vi "GetDecorationOwner.vi"(7 "VI Interpreter in":refnum<class "VI Interpreter.lvclass">, 8 "error in":errorcluster, 11 "Decoration in":refnum<class "Decoration.lvclass">) -> (0 "error out":errorcluster, 3 "Decoration out":refnum<class "Decoration.lvclass">, 4 "owner":string, 5 "VI Interpreter out":refnum<class "VI Interpreter.lvclass">)   [LabVIEW 2014, in "PythonConverter_GUI.lvclass"]
uses:
  PythonConverter_GUI.lvclass
  VI Interpreter/Classes/Decoration/Decoration.lvclass
  VI Interpreter/Classes/VI Interpreter/VI Interpreter.lvclass
  VI Interpreter/Classes/Generic/Generic.lvclass/Generic.ctl
  VI Interpreter/Classes/GObject/GObject.lvclass
  VI Interpreter/Classes/Tab/Tab.lvclass
  VI Interpreter/Classes/Generic/Generic.lvclass
  Parsing/Python Functions.lvlib
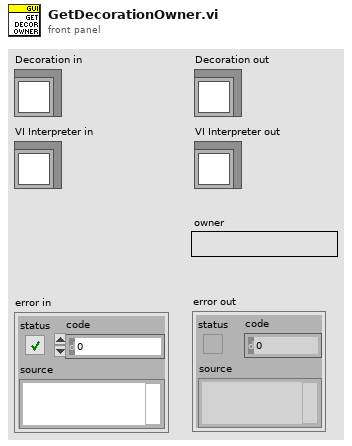
[diagram p1: front panel]
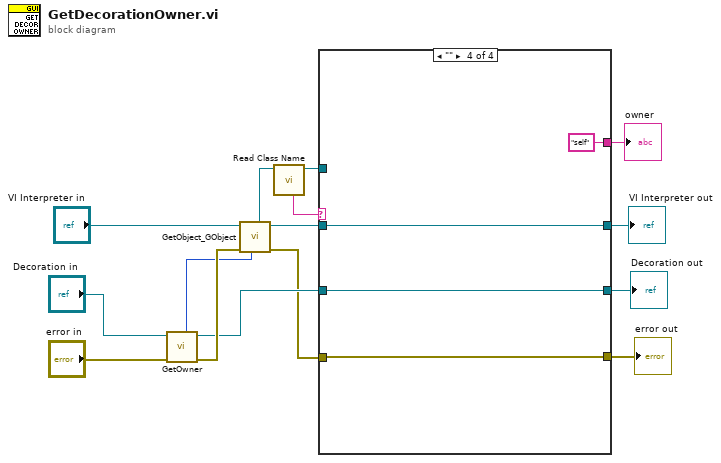
[diagram p0: block diagram]
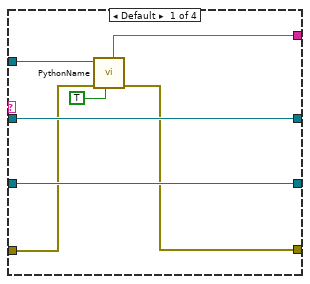
[diagram p2: hidden frame]
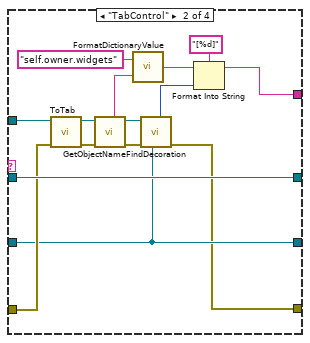
[diagram p3: hidden frame]
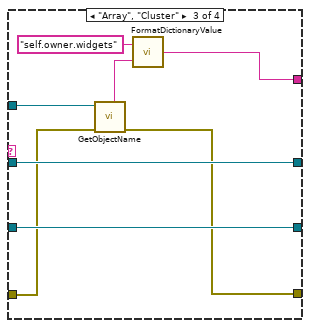
[diagram p4: hidden frame]
diagram:
  n1 = call-dynamic "GetOwner.vi"("error in"="error in", "GObject in"="Decoration in") -> ("error out"=w12:errorcluster, "GObject out"=w4:refnum<class "Decoration.lvclass">, "Owner"=w1:i32)  [unwired: 5 in]
  n2 = call "GetObject_GObject.vi"("UID"=w1, "error in"=w12, "VI Interpreter in"="VI Interpreter in") -> ("error out"=w2:errorcluster, "VI Interpreter out"=w8:refnum<class "VI Interpreter.lvclass">, "GObject"=w11:refnum<class "GObject.lvclass">)  [unwired: 3 in, 1 out]
  n3 = call "Read Class Name.vi"("Generic in"=w11) -> ("Generic out"=w9:refnum<class "GObject.lvclass">, "Class Name"=w10:string)  [unwired: 7 in]
  n4 = case shown="\"\"" w10 {
    tunnel: w9 -> [w22 w36 w40 _]
    tunnel: [w21 w24 w41 "self" ("python object")] -> w7
    tunnel: w8 -> [w19 w37 w45 w48]
    tunnel: [w19 w37 w45 w48] -> w6
    tunnel: [w18 w34 w44 w47] -> w5
    tunnel: w4 -> [w18 w34 w44 w47]
    tunnel: [w17 w23 w38 w46] -> w3
    tunnel: w2 -> [w16 w35 w39 w46]
    frame Default {
      n5 = call-dynamic "PythonName.vi"("add self"=TRUE, "error in"=w16, "GObject in"=w22) -> ("error out"=w17:errorcluster, "name"=w21:string)  [unwired: 5 in, 2 out]
    }
    frame "TabControl" {
      n6 = call "ToTab.vi"("error in"=w35, "Generic in"=w36) -> ("error out"=w32:errorcluster, "Tab out"=w33:refnum<class "Tab.lvclass">)  [unwired: 8 in]
      n7 = call-dynamic "GetObjectName.vi"("error in"=w32, "GObject in"=w33) -> ("error out"=w28:errorcluster, "GObject out"=w29:refnum<class "Tab.lvclass">, "Name"=w31:string)  [unwired: 5 in]
      n8 = call "FormatDictionaryValue.vi"("key"=w31, "dictionary"="self.owner.widgets") -> ("python object"=w26:string)
      n9 = call "FindDecoration.vi"("Decoration in"=w34, "error in"=w28, "Tab in"=w29) -> ("error out"=w23:errorcluster, "Tab index"=w27:i32)  [unwired: 4 in, 1 out]
      n10 = Format Into String(format string="[%d]", initial string=w26, w27) -> (resulting string=w24:string)  [unwired: 1 in, 1 out]
    }
    frame "Array", "Cluster" {
      n11 = call-dynamic "GetObjectName.vi"("error in"=w39, "GObject in"=w40) -> ("error out"=w38:errorcluster, "Name"=w43:string)  [unwired: 5 in, 1 out]
      n12 = call "FormatDictionaryValue.vi"("key"=w43, "dictionary"="self.owner.widgets") -> ("python object"=w41:string)
    }
    frame "" {
    }
  }
  "error out" <- w3
  "Decoration out" <- w5
  "owner" <- w7
  "VI Interpreter out" <- w6
